vi "EnvMillikInit.vi"(8 "error in (no error)":errorcluster, 10 "db connection in":T1, 11 "VISA Refnum in":refnum<visa-resource-name>) -> (0 "error out":errorcluster, 2 "db connection out":T1, 3 "VISA Refnum out":refnum<visa-resource-name>, 4 "sensor id array out":i32[](array[numeric]), 5 "channel array out":string[](array[string]))   [LabVIEW 2016]
uses:
  <vilib>/addons/database/Connection.llb/Conn ObjectReference.ctl
  <vilib>/addons/database/NI_Database_API.lvlib
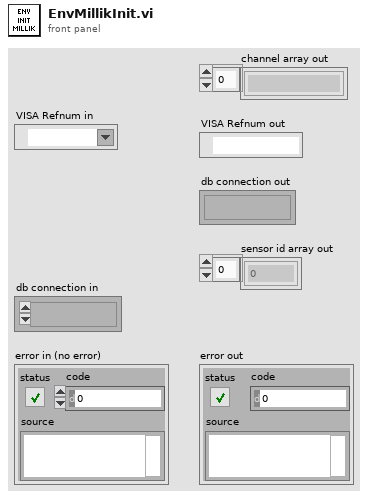
[diagram p1: front panel]
types:
  T1 = typedef "NI_Database_API.lvlib/Conn ObjectReference.ctl" = refnum<k1>
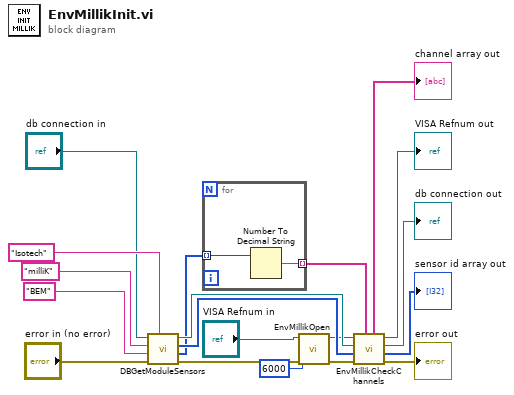
[diagram p0: block diagram]
diagram:
  n1 = call "DBGetModuleSensors.vi"("Module make"="Isotech", "error in (no error)"="error in (no error)", "Module loc"="BEM", "Module model"="milliK", "db connection in"="db connection in") -> ("error out"=w8:errorcluster, "sensor chan array"=w9:i32[], "sensor id array"=w16:i32[], "db connection out"=w17:T1)  [unwired: 3 in]
  n2 = for {
    tunnel: w9 -> [w21] mode=indexing
    tunnel: [w20] -> w15 mode=indexing
    n3 = Number To Decimal String(number=w21) -> (decimal integer string=w20:string)  [unwired: 1 in]
  }
  n4 = call "EnvMillikOpen.vi"("error in (no error)"=w8, "Read Timeout"=u32 6000, "VISA resource name"="VISA Refnum in") -> ("error out"=w10:errorcluster, "VISA resource name out"=w12:refnum<visa-resource-name>)  [unwired: 7 in]
  n5 = call "EnvMillikCheckChannels.vi"("channel array in"=w15, "error in (no error)"=w10, "sensor id array in"=w16, "db connection in"=w17, "VISA Refnum in"=w12) -> ("error out"=→"error out":errorcluster, "sensor id array out"=→"sensor id array out":i32[], "db connection out"=→"db connection out":T1, "VISA Refnum out"=→"VISA Refnum out":refnum<visa-resource-name>, "channel array out"=→"channel array out":string[])  [unwired: 2 in]
